vi "DeviceOff.vi"(8 "error in (no error)":errorcluster, 11 "NHRDCPower in":refnum<class "NHRDCPower.lvclass">) -> (0 "error out":errorcluster, 3 "NHRDCPower out":refnum<class "NHRDCPower.lvclass">)   [LabVIEW 2018, in "AcPwrPlugins.lvlib" / "NHRDCPower.lvclass"]
doc: "This VI disables the instruments output form either generating or receiving a signal."
uses:
  NHRDCPower.lvclass
  <instrlib>/NHRDCPowerModule/NHRDCPowerModule/NHRDCPowerModule.lvlib
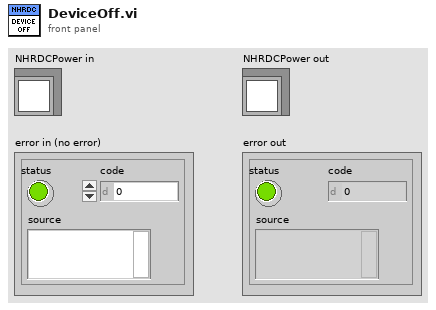
[diagram p1: front panel]
types:
  T1 = typedef "AcPwrPlugins.lvlib/NHRDCPower.lvclass/Device(s)Settings.ctl" = cluster{"Handle":string, "Name":string, "id query (Yes)":bool, "reset device (Yes)":bool, "Connected":bool, "Voltage Range (V)":dbl[], "Timing":cluster{"TimingOn":enum16{""}, "Hours":u32, "Minutes":u32, "Seconds":dbl, "CutoffVoltage":dbl}, "Initial Battery Detect Voltage (0)":sgl, "SafetySettings":cluster{"SetWatchDog":bool, "Voltage (V)":sgl, "Current (A)":sgl, "Power (W)":sgl, "Voltage Delay (s)":sgl, "Current Delay (s)":sgl, "Power Delay (s)":sgl}, "Options String":string, "Aperture Time (s)":sgl, "operating state (Off)":i32, "OutputSettings":cluster{"Voltage (V)":sgl, "Current (A)":sgl, "Resistance (Ohms)":sgl, "Power (W)":sgl, "Enable Voltage":bool, "Enable Current":bool, "Enable Resistance":bool, "Enable Power":bool, "Delay After (s)":sgl, "Wait Value (V, A, W)":sgl, "Enable Wait":bool, "Wait on Value":i32}[], "SlewRate":cluster{"Set Voltage Rate V/S":sgl, "Set Current Rate A/S":sgl, "Set Resistance Rate R/S":sgl, "Set Power Rate W/S":sgl}}[]
  T2 = cluster{"Voltage (V)":sgl, "Current (A)":sgl, "Resistance (Ohms)":sgl, "Power (W)":sgl, "Enable Voltage":bool, "Enable Current":bool, "Enable Resistance":bool, "Enable Power":bool, "Delay After (s)":sgl, "Wait Value (V, A, W)":sgl, "Enable Wait":bool, "Wait on Value":i32}[]
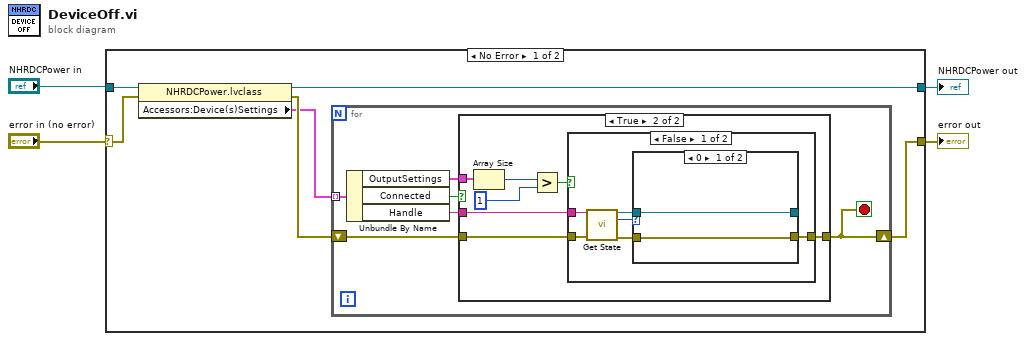
[diagram p0: block diagram]
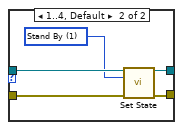
[diagram p3: hidden frame]
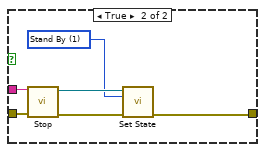
[diagram p4: hidden frame]
diagram:
  n1 = case shown="No Error" "error in (no error)" {
    selector: "error in (no error)" -> [w9 w45]
    tunnel: [w8 w45] -> w1
    tunnel: [w10 w44] -> w2
    tunnel: "NHRDCPower in" -> [w6 w44]
    frame No Error {
      n2 = property class="NHRDCPower.lvclass"(reference=w6, error in=w9) -> (reference out=w10:refnum<class "NHRDCPower.lvclass">, error out=w7:errorcluster, "Accessors:Device(s)Settings"=w5:T1)
      n3 = for {
        tunnel: w5 -> [w16] mode=indexing
        shift-right: [w14] -> w8
        shift-left: w7 -> [w15]
        stop <- w14 stop-if-true
        n4 = Unbundle By Name(w16) -> ("OutputSettings"=w11:T2, "Connected"=w12:bool, "Handle"=w13:string)
        n5 = case shown="True" w12 {
          tunnel: w15 -> [w17 w22]
          tunnel: [w17 w24] -> w14
          tunnel: w13 -> [_ w23]
          tunnel: w11 -> [_ w19]
          frame False {
          }
          frame True {
            n6 = Array Size(array=w19) -> (size(s)=w21:i32)
            n7 = Greater?(x=w21, y=1) -> (0:w18:bool)
            n8 = case shown="False" w18 {
              tunnel: [w30 w40] -> w24
              tunnel: w23 -> [w29 w42]
              tunnel: w22 -> [w28 w43]
              frame False {
                n9 = call <instrlib>:"Get State.vi"("instrument handle"=w29, "error in (no error)"=w28) -> ("instrument handle out"=w25:refnum<visa-resource-name>, "operating state"=w26:i32, "error out"=w27:errorcluster)  [unwired: 3 in, 8 out]
                n10 = case shown="0" w26 {
                  tunnel: [w32 w36] -> w30
                  tunnel: w27 -> [w32 w37]
                  tunnel: w25 -> [w31 w35]
                  tunnel: [w31 w33] -> _
                  frame 0 {
                  }
                  frame 1..4, Default {
                    w34 = 1 items=["Off", "Stand By", "Charge", "Discharge", "Battery Emulation"] ("operating state (Off)")
                    n11 = call <instrlib>:"Set State.vi"("instrument handle"=w35, "operating state (Off)"=w34, "error in (no error)"=w37) -> ("instrument handle out"=w33:refnum<visa-resource-name>, "error out"=w36:errorcluster)  [unwired: 11 in]
                  }
                }
              }
              frame True {
                w38 = 1 items=["Off", "Stand By", "Charge", "Discharge", "Battery Emulation"] ("operating state (Off)")
                n12 = call <instrlib>:"Stop.vi"("error in (no error)"=w43, "instrument handle"=w42) -> ("error out"=w41:errorcluster, "instrument handle out"=w39:refnum<visa-resource-name>)  [unwired: 8 in]
                n13 = call <instrlib>:"Set State.vi"("instrument handle"=w39, "operating state (Off)"=w38, "error in (no error)"=w41) -> ("error out"=w40:errorcluster)  [unwired: 11 in, 1 out]
              }
            }
          }
        }
      }
    }
    frame Error {
    }
  }
  "error out" <- w1
  "NHRDCPower out" <- w2
